vi "Lockin-4461 IV mode trigger and wait.vi"(8 "error in (no error)":errorcluster, 11 "Instrument.Lockin in":refnum<class "Instrument.Lockin.lvclass">) -> (0 "error out":errorcluster, 2 "AI Waveform":waveform(dbl)[](array[waveform]), 3 "Instrument.Lockin out":refnum<class "Instrument.Lockin.lvclass">)   [LabVIEW 2016, in "Instrument.Lockin.lvclass"]
uses:
  Instrument.Lockin.lvclass
  LockinDAQ/LockinDAQ.lvclass
  <vilib>/ErrorRing/Error Ring.xnode
  <vilib>/Utility/error.llb/Error Cluster From Error Code.vi
panel:
  in  "stop":bool
  out "timer (s)":dbl=1.2239999771118164
  # "This VI triggers the lockin and waits until the acquisition is complete"
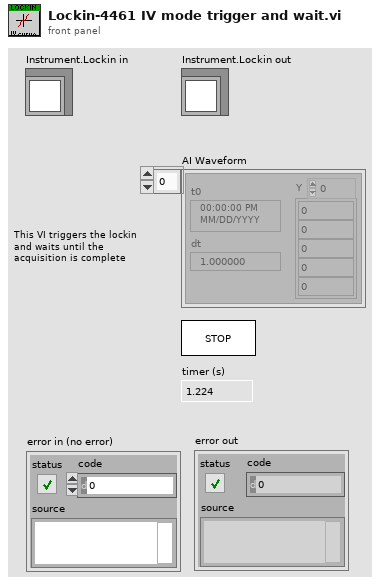
[diagram p1: front panel]
types:
  T1 = typedef "LockinDAQ.lvclass/AO-cluster.ctl" = cluster{"AO Amp (V)":T2, "AO DC (V)":T3, "AO f (Hz)":T4, "AO Phase (°)":T5, "Function":T6, "I+":bool[], "Sweeping":bool[]}
  T2 = typedef "LockinDAQ.lvclass/AO_Amp-array.ctl" = dbl[]
  T3 = typedef "LockinDAQ.lvclass/AO_DC-array.ctl" = dbl[]
  T4 = typedef "LockinDAQ.lvclass/AO_f-array.ctl" = dbl[]
  T5 = typedef "LockinDAQ.lvclass/AO_phi-array.ctl" = dbl[]
  T6 = typedef "LockinDAQ.lvclass/Function-array.ctl" = T7[]
  T7 = typedef "LockinDAQ.lvclass/Function-enum.ctl" = enum16{"Sine", "Triangle", "Square", "Sawtooth"}
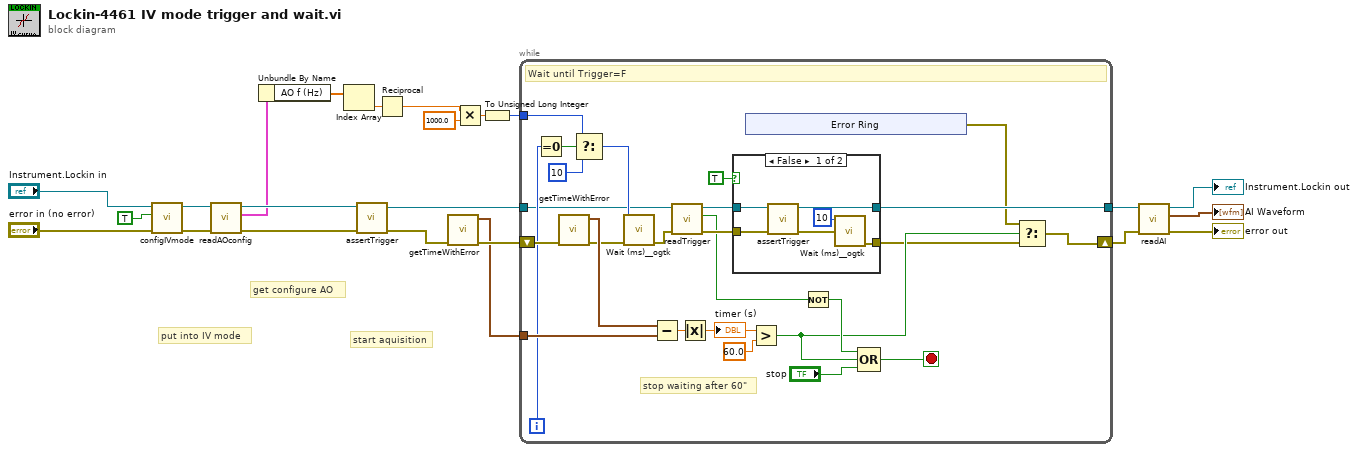
[diagram p0: block diagram]
diagram:
  # "start aquisition"
  # "get configure AO"
  # "put into IV mode"
  n1 = call "configIVmode.vi"("error in (no error)"="error in (no error)", "IV mode"=TRUE, "Instrument.Lockin in"="Instrument.Lockin in") -> ("error out"=w8:errorcluster, "Instrument.Lockin out"=w7:refnum<class "Instrument.Lockin.lvclass">)  [unwired: 7 in]
  n2 = call "readAOconfig.vi"("error in (no error)"=w8, "Instrument.Lockin in"=w7) -> ("error out"=w6:errorcluster, "AOconfig"=w3:T1, "Instrument.Lockin out"=w5:refnum<class "Instrument.Lockin.lvclass">)  [unwired: 7 in]
  n3 = Unbundle By Name(w3) -> ("AO f (Hz)"=w19:T4)
  n4 = Index Array(array=w19) -> (element=w18:dbl)  [unwired: 1 in]
  n5 = call "assertTrigger.vi"("error in (no error)"=w6, "Instrument.Lockin in"=w5) -> ("error out"=w4:errorcluster, "Instrument.Lockin out"=w10:refnum<class "Instrument.Lockin.lvclass">)  [unwired: 8 in]
  n6 = Reciprocal(x=w18) -> (1/x=w15:dbl)
  n7 = call "getTimeWithError.vi"("error in (no error)"=w4) -> ("error out"=w22:errorcluster, "seconds since 1Jan1904"=w21:timestamp)  [unwired: 9 in]
  n8 = Multiply(x=w15, y=1000.0) -> (x*y=w16:dbl)
  n9 = To Unsigned Long Integer(number=w16) -> (unsigned 32bit integer=w14:u32)
  n10 = while {
    shift-right: [w25] -> w2
    shift-left: w22 -> [w46]
    tunnel: w21 -> [w44]
    tunnel: w14 -> [w32]
    tunnel: [w30] -> w11
    tunnel: w10 -> [w28]
    i -> [w36]
    stop <- w42 stop-if-true
    # "stop waiting after 60\""
    # "Wait until Trigger=F"
    n11 = Equal To 0?(x=w36) -> (x = 0?=w35:bool)
    n12 = call "getTimeWithError.vi"("error in (no error)"=w46) -> ("error out"=w39:errorcluster, "seconds since 1Jan1904"=w45:timestamp)  [unwired: 9 in]
    n13 = Select(t=w32, s=w35, f=u32 10) -> (s? t:f=w33:u32)
    n14 = call <userlib>:"Wait (ms)__ogtk.vi"("error in (no error)"=w39, "milliseconds to wait"=w33) -> ("error out"=w38:errorcluster)  [unwired: 8 in, 1 out]
    n15 = Subtract(x=w45, y=w44) -> (x-y=w49:dbl)
    n16 = call "readTrigger.vi"("error in (no error)"=w38, "Instrument.Lockin"=w28) -> ("error out"=w41:errorcluster, "Trigger"=w31:bool, "Instrument.Lockin"=w29:refnum<class "Instrument.Lockin.lvclass">)  [unwired: 7 in]
    n17 = Absolute Value(x=w49) -> (abs(x)=w47:dbl)
    "timer (s)" <- w47
    n18 = case shown="False" TRUE {
      tunnel: w41 -> [w59 w61]
      tunnel: [w56 w61] -> w26
      tunnel: [w55 w60] -> w30
      tunnel: w29 -> [w54 w60]
      frame False {
        n19 = call "assertTrigger.vi"("error in (no error)"=w59, "Instrument.Lockin in"=w54) -> ("error out"=w57:errorcluster, "Instrument.Lockin out"=w55:refnum<class "Instrument.Lockin.lvclass">)  [unwired: 8 in]
        n20 = call <userlib>:"Wait (ms)__ogtk.vi"("error in (no error)"=w57, "milliseconds to wait"=u32 10) -> ("error out"=w56:errorcluster)  [unwired: 8 in, 1 out]
      }
      frame True {
      }
    }
    n21 = xnode "Error Ring"() -> ("error out"=w24:errorcluster)
    n22 = Greater?(x=w47, y=60.0) -> (0:w27:bool)
    n23 = Not(x=w31) -> (.not. x?=w43:bool)
    n24 = Compound Arithmetic op=OR(w43, w27, "stop") -> (w42:bool)
    n25 = Select(t=w24, s=w27, f=w26) -> (s? t:f=w25:errorcluster)
  }
  n26 = call "readAI.vi"("error in (no error)"=w2, "Instrument.Lockin in"=w11) -> ("error out"=→"error out":errorcluster, "AI Waveform"=→"AI Waveform":waveform(dbl)[], "Instrument.Lockin out"=→"Instrument.Lockin out":refnum<class "Instrument.Lockin.lvclass">)  [unwired: 7 in]
